vi "findneodevices.vi"(8 "error in (no error)":errorcluster) -> (0 "error out":errorcluster, 1 "pNumDevices":i32, 3 "NeoDevices {}":T1(array[cluster]) {"DeviceType" items=["NEODEVICE_BLUE"=1, "NEODEVICE_DW_VCAN"=4, "NEODEVICE_FIRE"=8, "NEODEVICE_VCAN3"=16, "NEODEVICE_YELLOW"=32, "NEODEVICE_ALL"=65535]})   [LabVIEW 2018]
doc: "This vi finds the available compatible devices on the network.\n\n<B>DeviceType</B>: device to find. multiple device types can be used by using the <B>logical OR</B> operator\n\n<B>Error In</B> : If error, then this call will be skipped and the error is passed through\n\n<B>NeoDevices {}</B> : the found devices array\n\n<B>pNumDevices</B> : number of devices found\n\n<B>Error Out</B> : returns the error produced by the call\n\n12/21/2010 1.0.0 jyg\n- initial release"
uses:
  icsneo40.dll
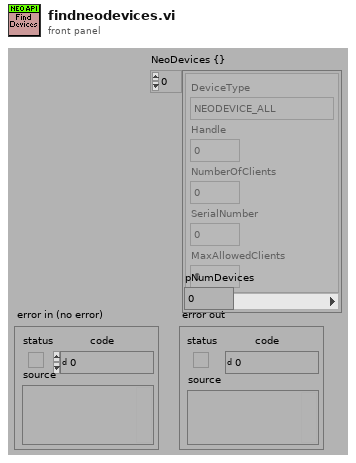
[diagram p1: front panel]
types:
  T1 = cluster{"DeviceType":i32, "Handle":i32, "NumberOfClients":i32, "SerialNumber":i32, "MaxAllowedClients":i32}[]
  T2 = cluster{"DeviceType":i32, "Handle":i32, "NumberOfClients":i32, "SerialNumber":i32, "MaxAllowedClients":i32}
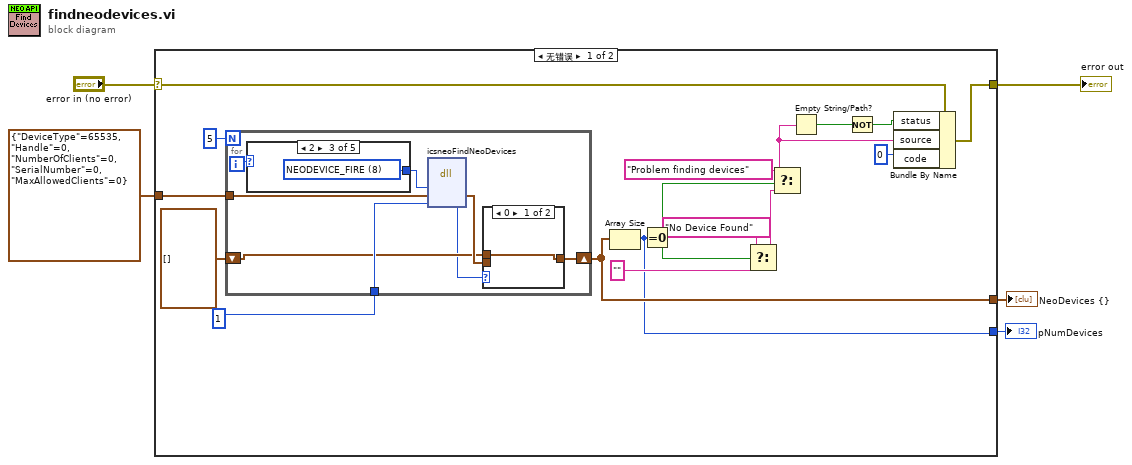
[diagram p0: block diagram]
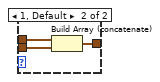
[diagram p2: hidden frame]
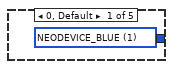
[diagram p3: hidden frame]
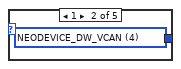
[diagram p4: hidden frame]
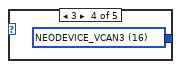
[diagram p5: hidden frame]
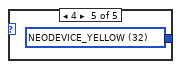
[diagram p6: hidden frame]
diagram:
  n1 = case shown="无错误" "error in (no error)" {
    selector: "error in (no error)" -> [w18 w40]
    tunnel: [w9 _] -> w3
    tunnel: [w19 w40] -> w5
    tunnel: [w6 _] -> w2
    tunnel: T2 {"DeviceType"=65535, "Handle"=0, "NumberOfClients"=0, "SerialNumber"=0, "MaxAllowedClients"=0} ("NeoDevice{}") -> [w13 _]
    frame No Error {
      n2 = for {
        N: 5 -> [_]
        tunnel: 1 -> [w30]
        tunnel: w13 -> [w29]
        shift-right: [w24] -> w9
        shift-left: T1 [] -> [w25]
        i -> [w28]
        n3 = case shown="2" w28 {
          tunnel: [w35 w36 w37 w38 w39] -> w27
          frame 0, Default {
            w35 = 1 items=["NEODEVICE_BLUE"=1, "NEODEVICE_DW_VCAN"=4, "NEODEVICE_FIRE"=8, "NEODEVICE_VCAN3"=16, "NEODEVICE_YELLOW"=32, "NEODEVICE_ALL"=65535] ("DeviceType")
          }
          frame 1 {
            w36 = 4 items=["NEODEVICE_BLUE"=1, "NEODEVICE_DW_VCAN"=4, "NEODEVICE_FIRE"=8, "NEODEVICE_VCAN3"=16, "NEODEVICE_YELLOW"=32, "NEODEVICE_ALL"=65535] ("DeviceType")
          }
          frame 2 {
            w37 = 8 items=["NEODEVICE_BLUE"=1, "NEODEVICE_DW_VCAN"=4, "NEODEVICE_FIRE"=8, "NEODEVICE_VCAN3"=16, "NEODEVICE_YELLOW"=32, "NEODEVICE_ALL"=65535] ("DeviceType")
          }
          frame 3 {
            w38 = 16 items=["NEODEVICE_BLUE"=1, "NEODEVICE_DW_VCAN"=4, "NEODEVICE_FIRE"=8, "NEODEVICE_VCAN3"=16, "NEODEVICE_YELLOW"=32, "NEODEVICE_ALL"=65535] ("DeviceType")
          }
          frame 4 {
            w39 = 32 items=["NEODEVICE_BLUE"=1, "NEODEVICE_DW_VCAN"=4, "NEODEVICE_FIRE"=8, "NEODEVICE_VCAN3"=16, "NEODEVICE_YELLOW"=32, "NEODEVICE_ALL"=65535] ("DeviceType")
          }
        }
        n4 = dll-call lib="icsneo40.dll" fn="icsneoFindNeoDevices"("DeviceTypes"=w27, w29, "pNumDevices"=w30) -> (w26:T2, "pNumDevices"=w23:i32)  [unwired: 4 in, 3 out]
        n5 = case shown="0" w23 {
          tunnel: w26 -> [_ w34]
          tunnel: w25 -> [w31 w33]
          tunnel: [w31 w32] -> w24
          frame 0 {
          }
          frame 1, Default {
            n6 = Build Array (concatenate)(w33, w34) -> (w32:T1)
          }
        }
      }
      n7 = Array Size(array=w9) -> (size(s)=w6:i32)
      n8 = Equal To 0?(x=w6) -> (x = 0?=w8:bool)
      n9 = Select(t="No Device Found", s=w8, f="") -> (s? t:f=w14:string)
      n10 = Select(t="Problem finding devices", s=w8, f=w14) -> (s? t:f=w17:string)
      n11 = Empty String/Path?(string/path=w17) -> (empty?=w21:bool)
      n12 = Not(x=w21) -> (.not. x?=w20:bool)
      n13 = Bundle By Name(cluster=w18, "status"=w20, "source"=w17, "code"=0) -> (w19:errorcluster)
    }
    frame Error {
    }
  }
  "error out" <- w5
  "NeoDevices {}" <- w3
  "pNumDevices" <- w2
